vi "esdaq_digitalDirection.vi"(2 "esdaqErrorInp":errorcluster, 3 "Value":bool, 4 "Channel":u8, 5 "esdaqPortInp":refnum<visa-resource-name>) -> (0 "esdaqErrorOut":errorcluster, 1 "esdaqPortOut":refnum<visa-resource-name>)   [LabVIEW 2019]
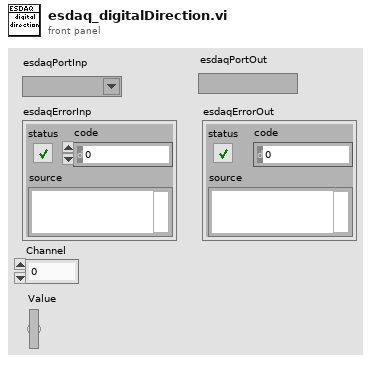
[diagram p1: front panel]
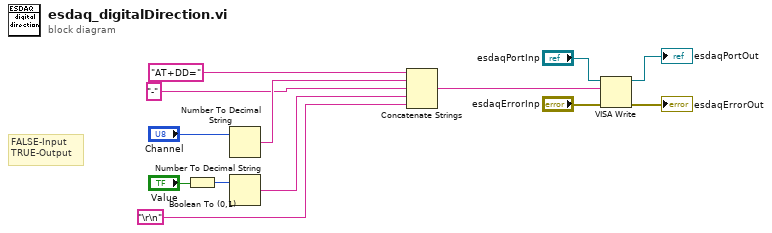
[diagram p0: block diagram]
diagram:
  # "FALSE-Input\nTRUE-Output"
  n1 = Boolean To (0,1)(Boolean="Value") -> (0, 1=w1:i16)
  n2 = Number To Decimal String(number="Channel") -> (decimal integer string=w11:string)  [unwired: 1 in]
  n3 = Number To Decimal String(number=w1) -> (decimal integer string=w9:string)  [unwired: 1 in]
  n4 = Concatenate Strings("AT+DD=", w11, "-", w9, "\r\n") -> (w7:string)
  n5 = VISA Write(VISA resource name="esdaqPortInp", write buffer=w7, error in (no error)="esdaqErrorInp") -> (VISA resource name out=→"esdaqPortOut":refnum<visa-resource-name>, error out=→"esdaqErrorOut":errorcluster)  [unwired: 1 out]
